vi "API Usage Examples.vi"() -> ()   [LabVIEW 2020, in "ase.example.lvlib"]
doc: "<B>A range of API usage examples for different scenarios.</B>"
uses:
  ase.example.lvlib
  ase/ase/ase.lvclass/ase.ctl
  ase/ase/Configuration.ctl
  ase/ase/Windows UTF8 Conversion Mode.ctl
  ase/ase/Standard Output.ctl
  ase/ase/Did Exit.ctl
  ase/ase/Event References.ctl
  ase/ase/Standard Error.ctl
  ase/ase/Merge Call Library Errors.vi
  ase/ase/Trim Whitespace.vi
  ase/ase/Check Shared Library Version.vi
  ase/ase/Start Call.vi/a70fc713-9ee9-4497-bede-7e71c94245f2.vi
  ase/ase/Write Data to Std In.vi
  ase/ase/Error Invalid ASE Handle.vi
  ase/ase/Error Internal Library Implementation Error.vi
  <vilib>/Utility/error.llb/Error Cluster From Error Code.vi
  ase/ase/ase.lvclass
  ase/ase/Write Line to Std In .vi
panel:
  out "Exit Code":i32
  out "error out":errorcluster
  out "Exit Code":i32
  out "error out":errorcluster
  out "Std Out":string caption="Std Out (regex split on numeric)"
  out "Exit Code":i32
  out "error out":errorcluster
  out "Std Out":string
  out "error out":errorcluster
  out "Std Out":string
  out "error out":errorcluster
  out "Std Out":string
  out "Exit Code":i32
  out "error out":errorcluster
  out "Std Out":string
  out "Exit Code":i32
  out "error out":errorcluster
  out "error out":errorcluster
  out "Exit Code":i32
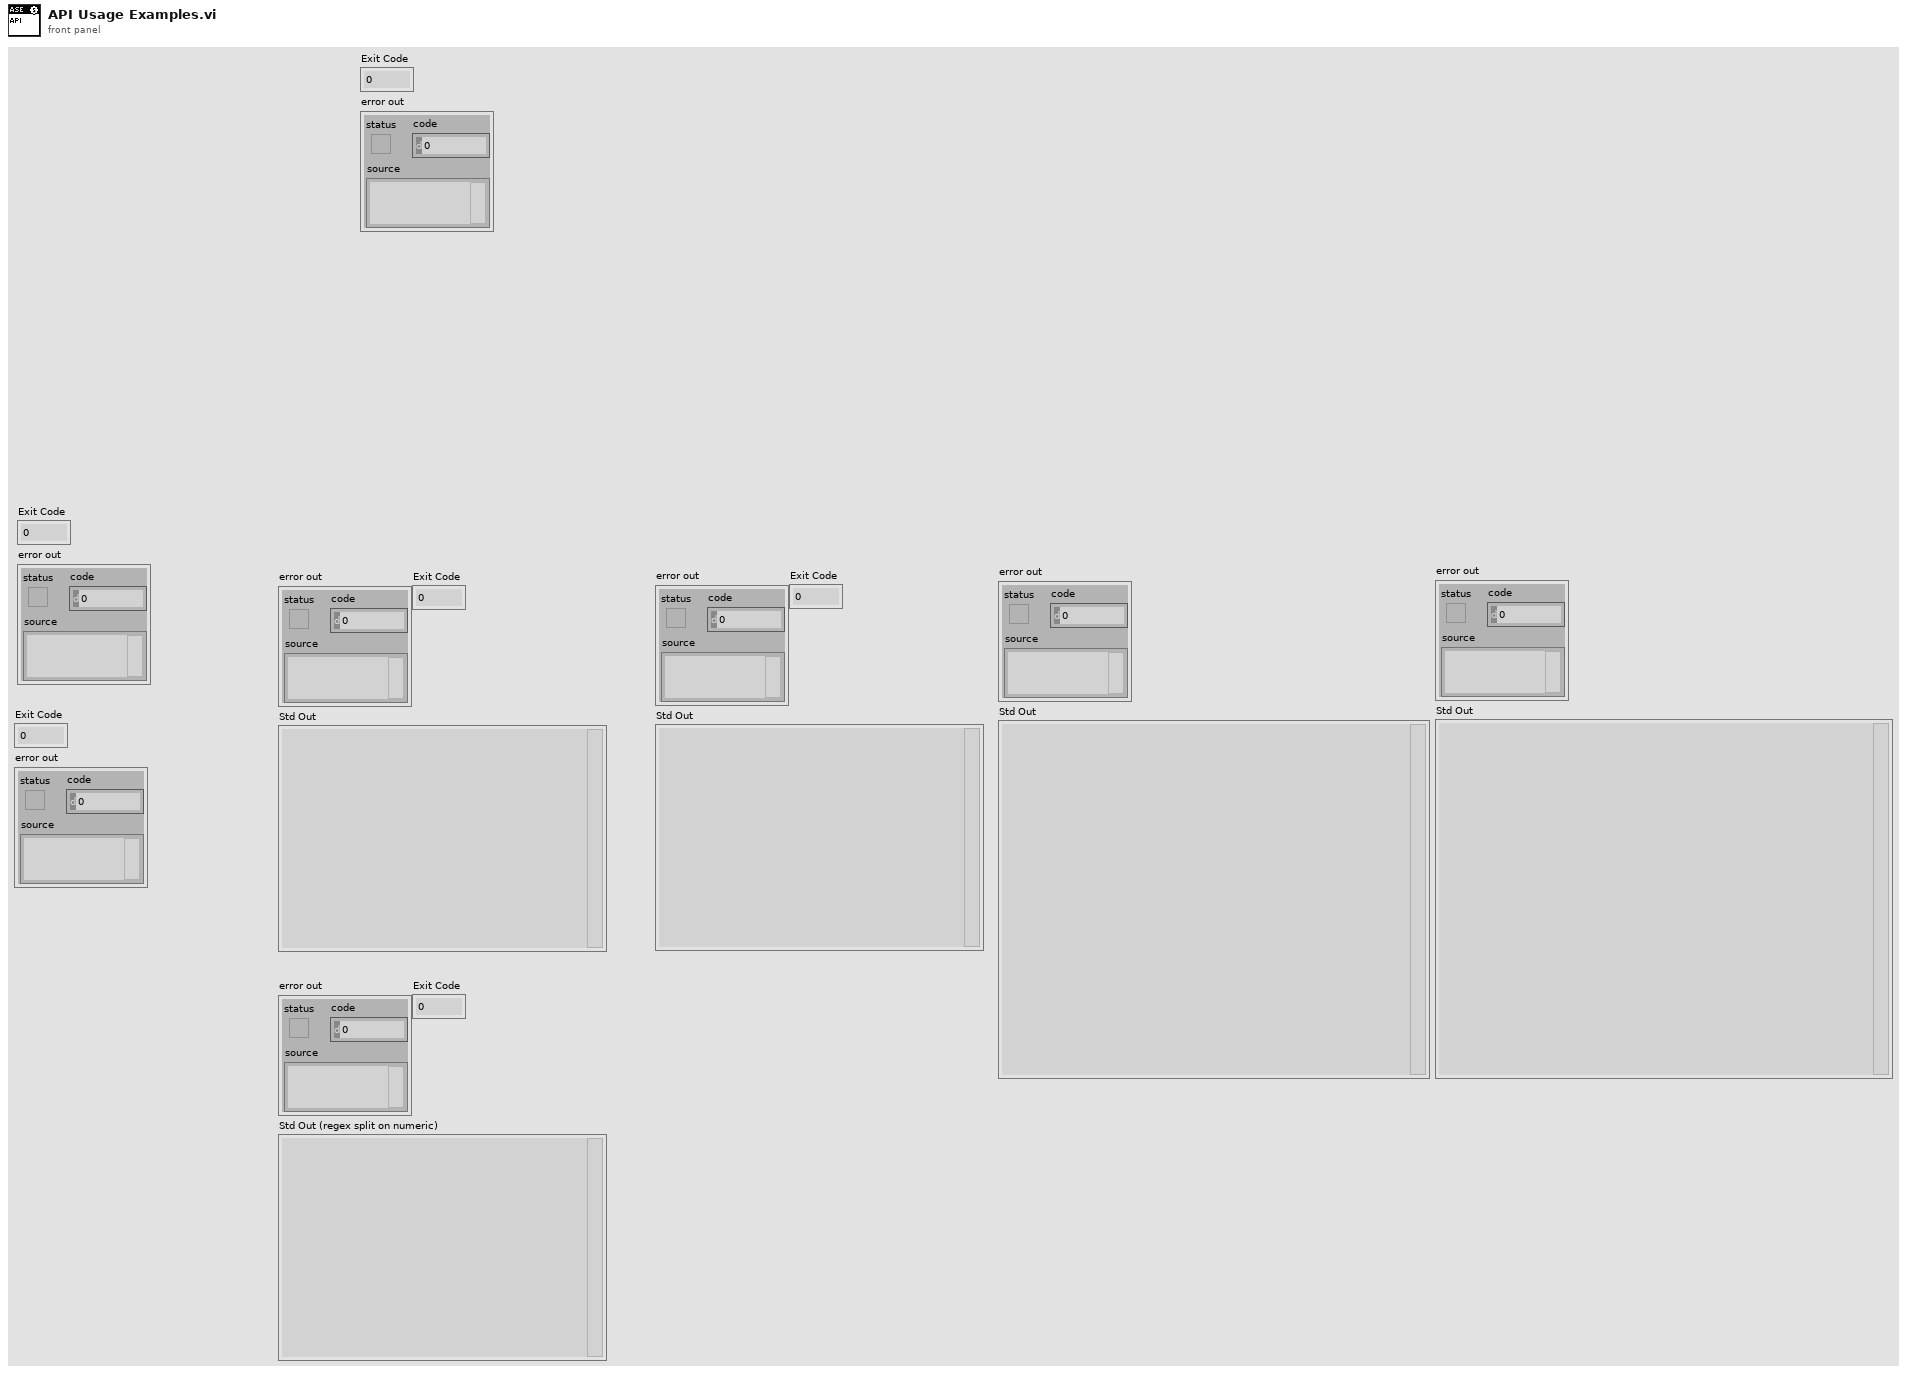
[diagram p1: front panel]
types:
  T1 = typedef "ase.lvlib/ase.lvclass/Configuration.ctl" = cluster{"Std Out Stream-Split RegExp Pattern":string, "Std Err Stream-Split RegExp Pattern":string, "ID":string, "Windows UTF8 Conversion":T2}
  T2 = typedef "ase.lvlib/ase.lvclass/Windows UTF8 Conversion Mode.ctl" = enum8{"None (Pass Through UTF8)", "To ACP Code Page", "To OEM Code Page"}
  T3 = typedef "ase.lvlib/ase.lvclass/Event References.ctl" = cluster{"Standard Output":refnum<user-event>, "Standard Error":refnum<user-event>, "Did Exit":refnum<user-event>}
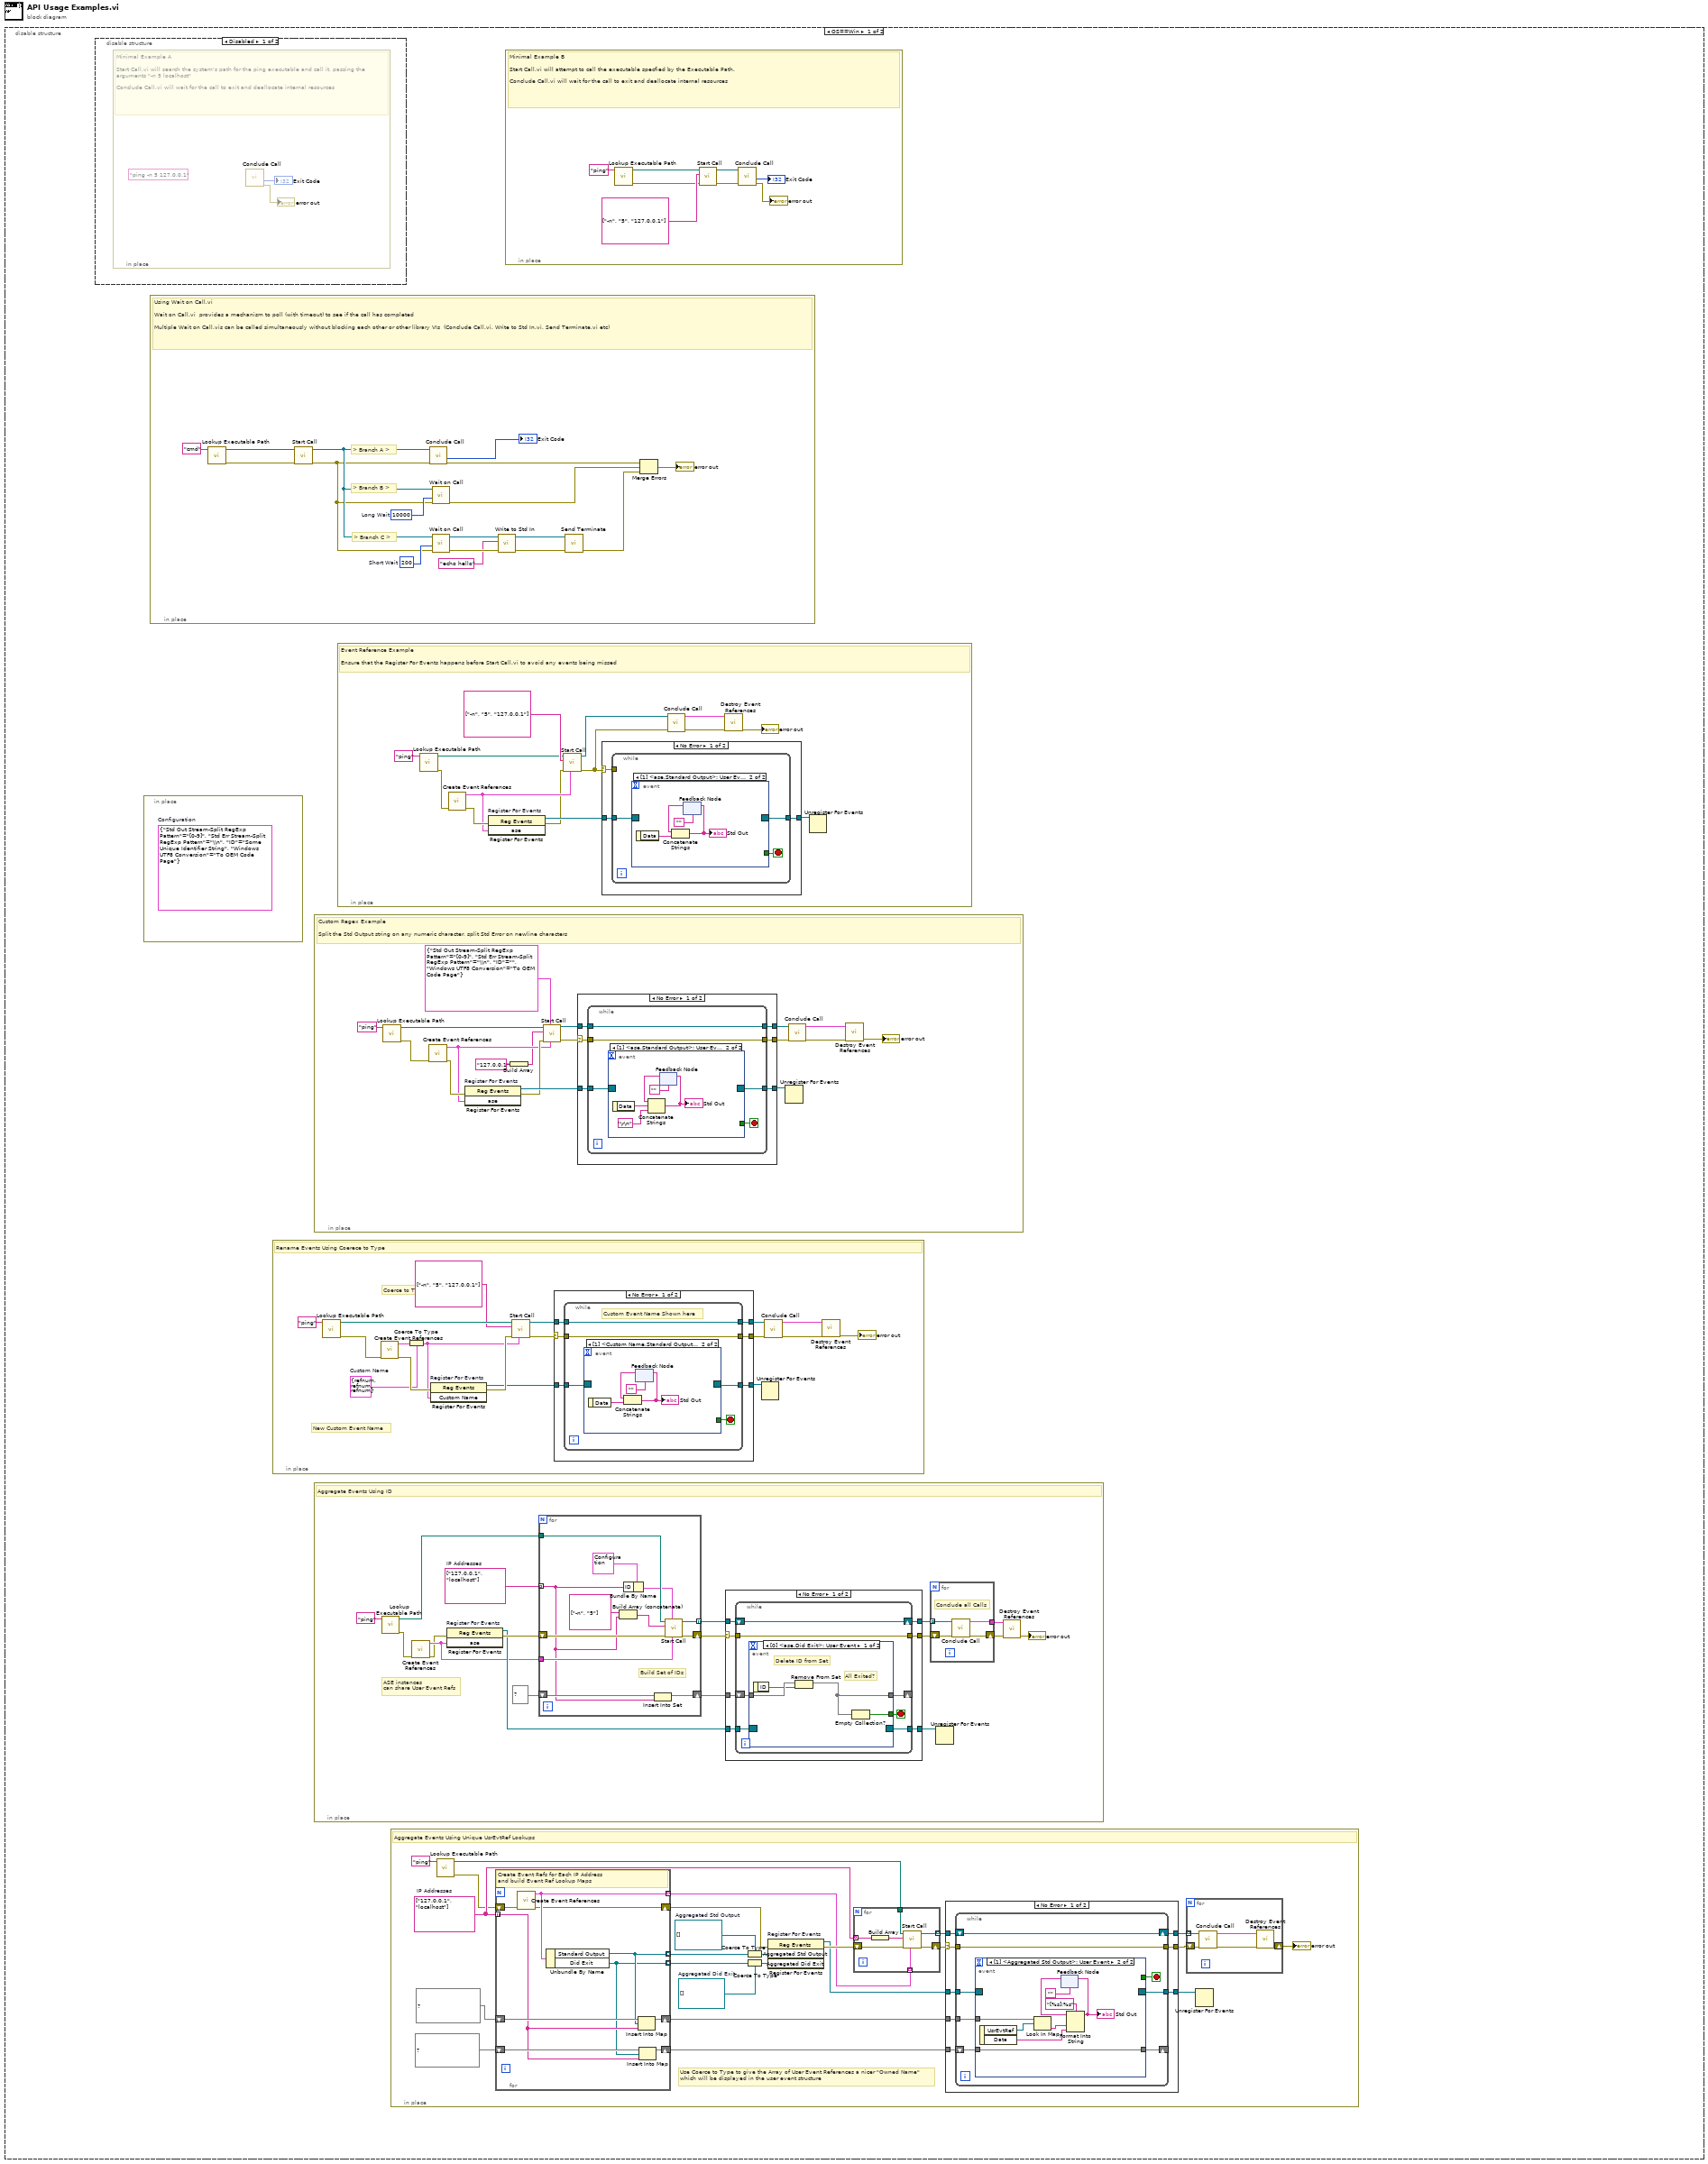
[diagram p0: block diagram]
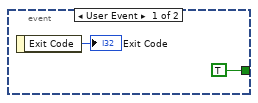
[diagram p3: hidden frame]
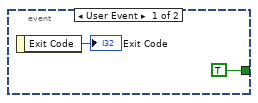
[diagram p5: hidden frame]
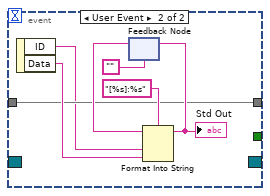
[diagram p7: hidden frame]
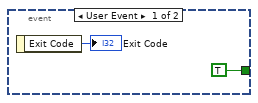
[diagram p9: hidden frame]
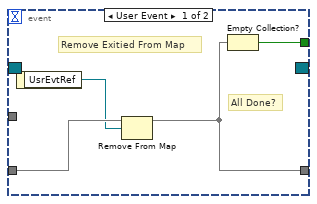
[diagram p11: hidden frame]
diagram:
  n1 = disable-structure shown="OS==Win" {
    frame condition #0 (active) {
      n2 = disable-structure shown="Disabled" {
        frame Disabled {
          n3 = in-place {
            w1 = "ping -n 5 127.0.0.1" ("cmd")
            # "Minimal Example A\n\nStart Call.vi will search the system's path for the ping executable and call it, passing the arguments \"-n 5 localhost\"\n\nConclude Call.vi will wait for the call to exit and deallocate internal resources"
            n4 = call "Conclude Call.vi"() -> ("error out"=→"error out":errorcluster, "Exit Code"=→"Exit Code":i32, "error in"=w5:errorcluster, "ASE Handle"=w4:refnum<class "ase.lvclass">)  [unwired: 7 in, 1 out]
          }
        }
        frame Enabled {
        }
      }
      n5 = in-place {
        (unwired) T1 {"Std Out Stream-Split RegExp Pattern"="[0-9]", "Std Err Stream-Split RegExp Pattern"="\\n", "ID"="Some Unique Identifier String", "Windows UTF8 Conversion"=enum."To OEM Code Page"}  # Configuration
      }
      n6 = in-place {
        w186 = 200  # Short Wait
        w187 = 10000  # Long Wait
        # "> Branch C >"
        # "> Branch B >"
        # "> Branch A >"
        # "Using Wait on Call.vi\n\nWait on Call.vi  provides a mechanism to poll (with timeout) to see if the call has completed\n\nMultiple Wait on Call.vis can be called simultaneously without blocking each other or other library VIs  (Conclude Call.vi, Write to Std In.vi, Send Terminate.vi etc)"
        n7 = call "Lookup Executable Path.vi"("Executable Name"="cmd") -> ("error out"=w173:errorcluster, "Path"=w172:path)  [unwired: 8 in, 1 out]
        n8 = call "Start Call.vi"("error in"=w173, "Executable Path"=w172) -> ("error out"=w177:errorcluster, "New ASE Handle"=w180:refnum<class "ase.lvclass">)  [unwired: 8 in]
        n9 = call "Conclude Call.vi"("error in"=w177, "ASE Handle"=w180) -> ("error out"=w179:errorcluster, "Exit Code"=→"Exit Code":i32)  [unwired: 7 in, 1 out]
        n10 = call "Wait on Call.vi"("error in"=w177, "Timeout (ms)"=w187, "ASE Handle"=w180) -> ("error out"=w176:errorcluster)  [unwired: 6 in, 2 out]
        n11 = call "Wait on Call.vi"("error in"=w177, "Timeout (ms)"=w186, "ASE Handle"=w180) -> ("error out"=w184:errorcluster, "ASE Handle Duplicate"=w185:refnum<class "ase.lvclass">)  [unwired: 6 in, 1 out]
        n12 = call-poly "Write to Std In.vi"("error in"=w184, "Input"="echo hello", "ASE Handle"=w185) -> ("error out"=w181:errorcluster, "ASE Handle Duplicate"=w182:refnum<class "ase.lvclass">)  [unwired: 6 in, 1 out]
        n13 = call "Send Terminate.vi"("error in"=w181, "ASE Handle"=w182) -> ("error out"=w175:errorcluster)  [unwired: 7 in, 2 out]
        n14 = Merge Errors(w179, w176, w175) -> (→"error out":errorcluster)
      }
      n15 = in-place {
        w139 = T3 {"Standard Output"=refnum, "Standard Error"=refnum, "Did Exit"=refnum}  # Custom Name
        # "New Custom Event Name"
        # "Coerce to Type"
        # "Rename Events Using Coerece to Type"
        n16 = call "Lookup Executable Path.vi"("Executable Name"="ping") -> ("error out"=w135:errorcluster, "Path"=w136:path)  [unwired: 8 in, 1 out]
        n17 = call "Create Event References.vi"("error in"=w135) -> ("error out"=w150:errorcluster, "ase"=w149:T3)  [unwired: 9 in]
        n18 = Coerce To Type(0:w149, 1:w139) -> (2:w138:T3)
        n19 = register-events "Register For Events"(error in=w150, w138) -> (reference out=w146:refnum<event-registration>, error out=w151:errorcluster)  [unwired: 1 in]
        n20 = call "Start Call.vi"("Event References"=w138, "error in"=w151, "Arguments (Default: Empty)"=string[] ["-n", "5", "127.0.0.1"], "Executable Path"=w136) -> ("error out"=w143:errorcluster, "New ASE Handle"=w148:refnum<class "ase.lvclass">)  [unwired: 6 in]
        n21 = case shown="No Error" w143 {
          selector: w143 -> [w155 w169]
          tunnel: w148 -> [w157 w170]
          tunnel: [w156 w170] -> w147
          tunnel: w146 -> [w154 w171]
          tunnel: [w153 w171] -> w145
          tunnel: [w152 w169] -> w144
          frame No Error {
            n22 = while {
              tunnel: w157 -> [w162]
              tunnel: [w162] -> w156
              tunnel: w155 -> [w159]
              tunnel: w154 -> [w161]
              tunnel: [w160] -> w153
              tunnel: [w159] -> w152
              stop <- w158 stop-if-true
              # "Custom Event Name Shown here"
              n23 = event shown="[1] <Custom Name.Standard Output>: User Event" {
                selector: w161 -> [_ _]
                dyn-events: [_ _] -> w160
                timeout: _ -> [_ _]
                tunnel: [TRUE _] -> w158
                event User Event {
                  n24 = event-data() -> ("Exit Code"=→"Exit Code":i32)  [unwired: 1 in]
                }
                event User Event {
                  n25 = event-data() -> ("Data"=w168:string)  [unwired: 1 in]
                  n26 = feedback #1("") -> (w166:string)
                  n27 = Concatenate Strings(w166, w168) -> (w167:string)
                  "Std Out" <- w167
                  n28 = feedback-in #1(w167) -> ()
                }
              }
            }
          }
          frame Error {
          }
        }
        n29 = Unregister For Events(event registration refnum=w145) -> ()  [unwired: 1 in, 1 out]
        n30 = call "Conclude Call.vi"("error in"=w144, "ASE Handle"=w147) -> ("error out"=w142:errorcluster, "Event References"=w141:T3)  [unwired: 7 in, 1 out]
        n31 = call "Destroy Event References.vi"("error in"=w142, "Event References"=w141) -> ("error out"=→"error out":errorcluster)  [unwired: 9 in]
      }
      n32 = in-place {
        w82 = string[] ["127.0.0.1", "localhost"]  # IP Addresses
        # "ASE instances\ncan share User Event Refs"
        # "Aggregate Events Using ID"
        n33 = call "Lookup Executable Path.vi"("Executable Name"="ping") -> ("error out"=w74:errorcluster, "Path"=w72:path)  [unwired: 8 in, 1 out]
        n34 = call "Create Event References.vi"("error in"=w74) -> ("error out"=w73:errorcluster, "ase"=w81:T3)  [unwired: 9 in]
        n35 = register-events "Register For Events"(error in=w73, w81) -> (reference out=w86:refnum<event-registration>, error out=w89:errorcluster)  [unwired: 1 in]
        n36 = for {
          tunnel: [w99] -> w88 mode=indexing
          shift-right: [w98] -> w83
          shift-left: w89 -> [w100]
          tunnel: w81 -> [w97]
          tunnel: w82 -> [w91] mode=indexing
          shift-right: [w96] -> w79
          shift-left: set{string} {} ("Size: 0") -> [w95]
          tunnel: w72 -> [w101]
          # "Build Set of IDs"
          # "Use IP Address as ID"
          n37 = Build Array (concatenate)(string[] ["-n", "5"], w91) -> (w90:string[])
          n38 = Bundle By Name(cluster=T1 {"Std Out Stream-Split RegExp Pattern"="\\n", "Std Err Stream-Split RegExp Pattern"="\\n", "ID"="", "Windows UTF8 Conversion"=enum."To OEM Code Page"} ("Configuration (Default)"), "ID"=w91) -> (w93:T1)
          n39 = Insert Into Set(10:w91, 11:w95) -> (3:w96:set{string})  [unwired: 1 out]
          n40 = call "Start Call.vi"("Event References"=w97, "Configuration (Default)"=w93, "error in"=w100, "Arguments (Default: Empty)"=w90, "Executable Path"=w101) -> ("error out"=w98:errorcluster, "New ASE Handle"=w99:refnum<class "ase.lvclass">)  [unwired: 5 in]
        }
        n41 = case shown="No Error" w83 {
          selector: w83 -> [w106 w127]
          tunnel: w88 -> [w108 w128]
          tunnel: [w107 w128] -> w87
          tunnel: w86 -> [w105 w129]
          tunnel: [w104 w129] -> w85
          tunnel: [w103 w127] -> w84
          tunnel: w79 -> [w102 _]
          frame No Error {
            n42 = while {
              tunnel: w106 -> [w112]
              tunnel: w105 -> [w114]
              tunnel: [w113] -> w104
              tunnel: [w112] -> w103
              shift-right: [w109] -> _
              shift-left: w102 -> [w110]
              shift-right: [w115] -> w107
              shift-left: w108 -> [w115]
              stop <- w111 stop-if-true
              n43 = event shown="[0] <ase.Did Exit>: User Event" {
                selector: w114 -> [_ _]
                dyn-events: [_ _] -> w113
                timeout: _ -> [_ _]
                tunnel: [w118 _] -> w111
                tunnel: w110 -> [w119 w121]
                tunnel: [w117 w121] -> w109
                event User Event {
                  # "All Exited?"
                  # "Delete ID from Set"
                  n44 = event-data() -> ("ID"=w116:string)  [unwired: 1 in]
                  n45 = Remove From Set(10:w116, 11:w119) -> (3:w117:set{string})  [unwired: 1 out]
                  n46 = Empty Collection?(1:w117) -> (0:w118:bool)
                }
                event User Event {
                  n47 = event-data() -> ("ID"=w120:string, "Data"=w122:string)  [unwired: 1 in]
                  n48 = feedback #2("") -> (w125:string)
                  n49 = Format Into String(format string="[%s]:%s", initial string=w125, w120, w122) -> (resulting string=w124:string)  [unwired: 1 in, 1 out]
                  "Std Out" <- w124
                  n50 = feedback-in #2(w124) -> ()
                }
              }
            }
          }
          frame Error {
          }
        }
        n51 = for {
          tunnel: w87 -> [w133] mode=indexing
          shift-right: [w130] -> w76
          shift-left: w84 -> [w132]
          tunnel: [w131] -> w78
          # "Conclude all Calls"
          n52 = call "Conclude Call.vi"("error in"=w132, "ASE Handle"=w133) -> ("error out"=w130:errorcluster, "Event References"=w131:T3)  [unwired: 7 in, 1 out]
        }
        n53 = Unregister For Events(event registration refnum=w85) -> ()  [unwired: 1 in, 1 out]
        n54 = call "Destroy Event References.vi"("error in"=w76, "Event References"=w78) -> ("error out"=→"error out":errorcluster)  [unwired: 9 in]
      }
      n55 = in-place {
        # "Custom Regex Example\n\nSplit the Std Output string on any numeric character, split Std Error on newline characters"
        n56 = call "Lookup Executable Path.vi"("Executable Name"="ping") -> ("error out"=w13:errorcluster, "Path"=w15:path)  [unwired: 8 in, 1 out]
        n57 = call "Create Event References.vi"("error in"=w13) -> ("error out"=w23:errorcluster, "ase"=w9:T3)  [unwired: 9 in]
        n58 = register-events "Register For Events"(error in=w23, w9) -> (reference out=w21:refnum<event-registration>, error out=w10:errorcluster)  [unwired: 1 in]
        n59 = Build Array("127.0.0.1" ("String")) -> (w6:string[])
        n60 = call "Start Call.vi"("Event References"=w9, "Configuration (Default)"=T1 {"Std Out Stream-Split RegExp Pattern"="[0-9]", "Std Err Stream-Split RegExp Pattern"="\\n", "ID"="", "Windows UTF8 Conversion"=enum."To OEM Code Page"}, "error in"=w10, "Arguments (Default: Empty)"=w6, "Executable Path"=w15) -> ("error out"=w11:errorcluster, "New ASE Handle"=w12:refnum<class "ase.lvclass">)  [unwired: 5 in]
        n61 = case shown="No Error" w11 {
          selector: w11 -> [w27 w42]
          tunnel: w12 -> [w29 w43]
          tunnel: [w28 w43] -> w22
          tunnel: w21 -> [w26 w44]
          tunnel: [w25 w44] -> w20
          tunnel: [w24 w42] -> w19
          frame No Error {
            n62 = while {
              tunnel: w29 -> [w34]
              tunnel: [w34] -> w28
              tunnel: w27 -> [w31]
              tunnel: w26 -> [w33]
              tunnel: [w32] -> w25
              tunnel: [w31] -> w24
              stop <- w30 stop-if-true
              n63 = event shown="[1] <ase.Standard Output>: User Event" {
                selector: w33 -> [_ _]
                dyn-events: [_ _] -> w32
                timeout: _ -> [_ _]
                tunnel: [TRUE _] -> w30
                event User Event {
                  n64 = event-data() -> ("Exit Code"=→"Exit Code":i32)  [unwired: 1 in]
                }
                event User Event {
                  n65 = event-data() -> ("Data"=w38:string)  [unwired: 1 in]
                  n66 = feedback #3("") -> (w40:string)
                  n67 = Concatenate Strings(w40, w38, "\r\n" ("string")) -> (w41:string)
                  "Std Out" <- w41
                  n68 = feedback-in #3(w41) -> ()
                }
              }
            }
          }
          frame Error {
          }
        }
        n69 = Unregister For Events(event registration refnum=w20) -> ()  [unwired: 1 in, 1 out]
        n70 = call "Conclude Call.vi"("error in"=w19, "ASE Handle"=w22) -> ("error out"=w18:errorcluster, "Event References"=w17:T3)  [unwired: 7 in, 1 out]
        n71 = call "Destroy Event References.vi"("error in"=w18, "Event References"=w17) -> ("error out"=→"error out":errorcluster)  [unwired: 9 in]
      }
      n72 = in-place {
        # "Event Reference Example\n\nEnsure that the Register For Events happens before Start Call.vi to avoid any events being missed"
        n73 = call "Lookup Executable Path.vi"("Executable Name"="ping") -> ("error out"=w47:errorcluster, "Path"=w51:path)  [unwired: 8 in, 1 out]
        n74 = call "Create Event References.vi"("error in"=w47) -> ("error out"=w58:errorcluster, "ase"=w49:T3)  [unwired: 9 in]
        n75 = register-events "Register For Events"(error in=w58, w49) -> (reference out=w57:refnum<event-registration>, error out=w48:errorcluster)  [unwired: 1 in]
        n76 = call "Start Call.vi"("Event References"=w49, "error in"=w48, "Arguments (Default: Empty)"=string[] ["-n", "5", "127.0.0.1"], "Executable Path"=w51) -> ("error out"=w45:errorcluster, "New ASE Handle"=w46:refnum<class "ase.lvclass">)  [unwired: 6 in]
        n77 = case shown="No Error" w45 {
          selector: w45 -> [w61 _]
          tunnel: w57 -> [w60 w71]
          tunnel: [w59 w71] -> w56
          frame No Error {
            n78 = while {
              tunnel: w61 -> [_]
              tunnel: w60 -> [w64]
              tunnel: [w63] -> w59
              stop <- w62 stop-if-true
              n79 = event shown="[1] <ase.Standard Output>: User Event" {
                selector: w64 -> [_ _]
                dyn-events: [_ _] -> w63
                timeout: _ -> [_ _]
                tunnel: [TRUE _] -> w62
                event User Event {
                  n80 = event-data() -> ("Exit Code"=→"Exit Code":i32)  [unwired: 1 in]
                }
                event User Event {
                  n81 = event-data() -> ("Data"=w70:string)  [unwired: 1 in]
                  n82 = feedback #4("") -> (w68:string)
                  n83 = Concatenate Strings(w68, w70) -> (w69:string)
                  "Std Out" <- w69
                  n84 = feedback-in #4(w69) -> ()
                }
              }
            }
          }
          frame Error {
          }
        }
        n85 = call "Conclude Call.vi"("error in"=w45, "ASE Handle"=w46) -> ("error out"=w55:errorcluster, "Event References"=w54:T3)  [unwired: 7 in, 1 out]
        n86 = call "Destroy Event References.vi"("error in"=w55, "Event References"=w54) -> ("error out"=→"error out":errorcluster)  [unwired: 9 in]
        n87 = Unregister For Events(event registration refnum=w56) -> ()  [unwired: 1 in, 1 out]
      }
      n88 = in-place {
        w193 = string[] ["127.0.0.1", "localhost"]  # IP Addresses
        w195 = refnum<user-event>[] []  # Aggregated Did Exit
        w194 = refnum<user-event>[] []  # Aggregated Std Output
        # "Use Coerce to Type to give the Array of User Event References a nicer \"Owned Name\"\nwhich will be displayed in the user event structure"
        # "Aggregate Events Using Unique UsrEvtRef Lookups"
        n89 = call "Lookup Executable Path.vi"("Executable Name"="ping") -> ("error out"=w191:errorcluster, "Path"=w189:path)  [unwired: 8 in, 1 out]
        n90 = for {
          tunnel: w193 -> [w228] mode=indexing
          shift-right: [w232] -> w200
          shift-left: map{refnum<user-event>, string} {} ("map out") -> [w233]
          shift-right: [w230] -> w199
          shift-left: map{refnum<user-event>, string} {} ("set out") -> [w229]
          tunnel: [w234] -> w201 mode=indexing
          tunnel: [w231] -> w203 mode=indexing
          tunnel: [w227] -> w202 mode=indexing
          shift-right: [w225] -> w190
          shift-left: w191 -> [w226]
          # "Create Event Refs for Each IP Address\nand build Event Ref Lookup Maps"
          n91 = call "Create Event References.vi"("error in"=w226) -> ("error out"=w225:errorcluster, "ase"=w234:T3)  [unwired: 9 in]
          n92 = Unbundle By Name(w234) -> ("Standard Output"=w231:refnum<user-event>, "Did Exit"=w227:refnum<user-event>)
          n93 = Insert Into Map(map in=w233, key=w231, value=w228) -> (map out=w232:map{refnum<user-event>, string})  [unwired: 2 out]
          n94 = Insert Into Map(map in=w229, key=w227, value=w228) -> (map out=w230:map{refnum<user-event>, string})  [unwired: 2 out]
        }
        n95 = Coerce To Type(0:w203, 1:w194) -> (2:w197:refnum<user-event>[])
        n96 = Coerce To Type(0:w202, 1:w195) -> (2:w196:refnum<user-event>[])
        n97 = register-events "Register For Events"(error in=w190, w197, w196) -> (reference out=w209:refnum<event-registration>, error out=w212:errorcluster)  [unwired: 1 in]
        n98 = for {
          tunnel: [w223] -> w211 mode=indexing
          shift-right: [w222] -> w206
          shift-left: w212 -> [w224]
          tunnel: w201 -> [w221] mode=indexing
          tunnel: w193 -> [w220] mode=indexing
          tunnel: w189 -> [w218]
          n99 = Build Array(w220) -> (w219:string[])
          n100 = call "Start Call.vi"("Event References"=w221, "error in"=w224, "Arguments (Default: Empty)"=w219, "Executable Path"=w218) -> ("error out"=w222:errorcluster, "New ASE Handle"=w223:refnum<class "ase.lvclass">)  [unwired: 6 in]
        }
        n101 = case shown="No Error" w206 {
          selector: w206 -> [w240 w264]
          tunnel: w211 -> [w242 w265]
          tunnel: [w241 w265] -> w210
          tunnel: w209 -> [w239 w266]
          tunnel: [w238 w266] -> w208
          tunnel: [w237 w264] -> w207
          tunnel: w200 -> [w236 _]
          tunnel: w199 -> [w235 _]
          frame No Error {
            n102 = while {
              tunnel: w240 -> [w247]
              tunnel: w239 -> [w249]
              tunnel: [w248] -> w238
              tunnel: [w247] -> w237
              tunnel: w236 -> [w245]
              shift-right: [w243] -> _
              shift-left: w235 -> [w244]
              shift-right: [w250] -> w241
              shift-left: w242 -> [w250]
              stop <- w246 stop-if-true
              n103 = event shown="[1] <Aggregated Std Output>: User Event" {
                selector: w249 -> [_ _]
                dyn-events: [_ _] -> w248
                timeout: _ -> [_ _]
                tunnel: [w252 _] -> w246
                tunnel: w245 -> [_ w262]
                tunnel: w244 -> [w254 w256]
                tunnel: [w251 w256] -> w243
                event User Event {
                  # "All Done?"
                  # "Remove Exitied From Map"
                  n104 = event-data() -> ("UsrEvtRef"=w253:refnum<user-event>)  [unwired: 1 in]
                  n105 = Remove From Map(10:w253, 11:w254) -> (3:w251:map{refnum<user-event>, string})  [unwired: 2 out]
                  n106 = Empty Collection?(1:w251) -> (0:w252:bool)
                }
                event User Event {
                  n107 = event-data() -> ("UsrEvtRef"=w261:refnum<user-event>, "Data"=w255:string)  [unwired: 1 in]
                  n108 = Look In Map(map=w262, key=w261) -> (value=w260:string)  [unwired: 1 in, 1 out]
                  n109 = feedback #5("") -> (w259:string)
                  n110 = Format Into String(format string="[%s]:%s", initial string=w259, w260, w255) -> (resulting string=w258:string)  [unwired: 1 in, 1 out]
                  "Std Out" <- w258
                  n111 = feedback-in #5(w258) -> ()
                }
              }
            }
          }
          frame Error {
          }
        }
        n112 = for {
          tunnel: w210 -> [w217] mode=indexing
          shift-right: [w213] -> w205
          shift-left: w207 -> [w216]
          n113 = call "Conclude Call.vi"("error in"=w216, "ASE Handle"=w217) -> ("error out"=w215:errorcluster, "Event References"=w214:T3)  [unwired: 7 in, 1 out]
          n114 = call "Destroy Event References.vi"("error in"=w215, "Event References"=w214) -> ("error out"=w213:errorcluster)  [unwired: 9 in]
        }
        "error out" <- w205
        n115 = Unregister For Events(event registration refnum=w208) -> ()  [unwired: 1 in, 1 out]
      }
      n116 = in-place {
        # "Minimal Example B\n\nStart Call.vi will attempt to call the executable specfied by the Executable Path.\n\nConclude Call.vi will wait for the call to exit and deallocate internal resources"
        n117 = call "Lookup Executable Path.vi"("Executable Name"="ping") -> ("error out"=w268:errorcluster, "Path"=w269:path)  [unwired: 8 in, 1 out]
        n118 = call "Start Call.vi"("error in"=w268, "Arguments (Default: Empty)"=string[] ["-n", "5", "127.0.0.1"], "Executable Path"=w269) -> ("error out"=w274:errorcluster, "New ASE Handle"=w273:refnum<class "ase.lvclass">)  [unwired: 7 in]
        n119 = call "Conclude Call.vi"("error in"=w274, "ASE Handle"=w273) -> ("error out"=→"error out":errorcluster, "Exit Code"=→"Exit Code":i32)  [unwired: 7 in, 1 out]
      }
    }
    frame condition #1 {
      # "These examples will work on other platforms but the ping executable needs to be supplied a \"ping count\"  with option -\"c\"  instead of option \"-n\""
    }
  }
